vi "Angle Converter- Degrees to Unit Circle Radians.vi"(11 "Angle in \nHeading \nFormat":T1 format="%05.1f") -> (3 "Angle in \nUnit Circle\nRadians":dbl)   [LabVIEW 2011]
doc: "Converts angles in heading format (clockwise degrees with North = 0) to unit circle radians (counterclockwise, East = positive X direction = 0)\nUse this before applying trigonometric functions to headings."
uses:
  2 Typedefs/heading.ctl
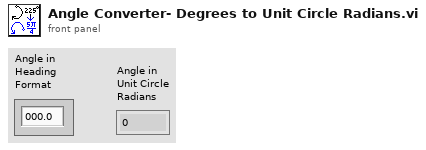
[diagram p1: front panel]
types:
  T1 = typedef "heading.ctl" = dbl
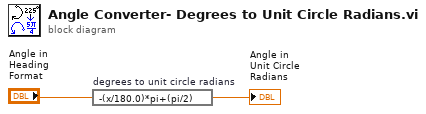
[diagram p0: block diagram]
diagram:
  n1 = expression code="-(x/180.0)*pi+(pi/2)" "degrees to unit circle radians"("Angle in \nHeading \nFormat") -> (→"Angle in \nUnit Circle\nRadians":T1)
